vi "delay stage BBD301.vi"() -> ()   [LabVIEW 2024]
uses:
  C:/Users/QLM-CCD/Desktop/Pump probe/Kinesis/Thorlabs.MotionControl.Benchtop.BrushlessMotorCLI.dll
  Kinesis/Thorlabs.MotionControl.Benchtop.BrushlessMotorCLI.dll
  C:/Users/QLM-CCD/Desktop/Pump probe/Kinesis/Thorlabs.MotionControl.Controls.dll
  Kinesis/Thorlabs.MotionControl.Controls.dll
panel:
  in  "end poisition (mm)":dbl
  in  "stop":bool
  out "Position (micrometer)":i32
  in  "BenchtopBrushlessControl":refnum<k24>(container)
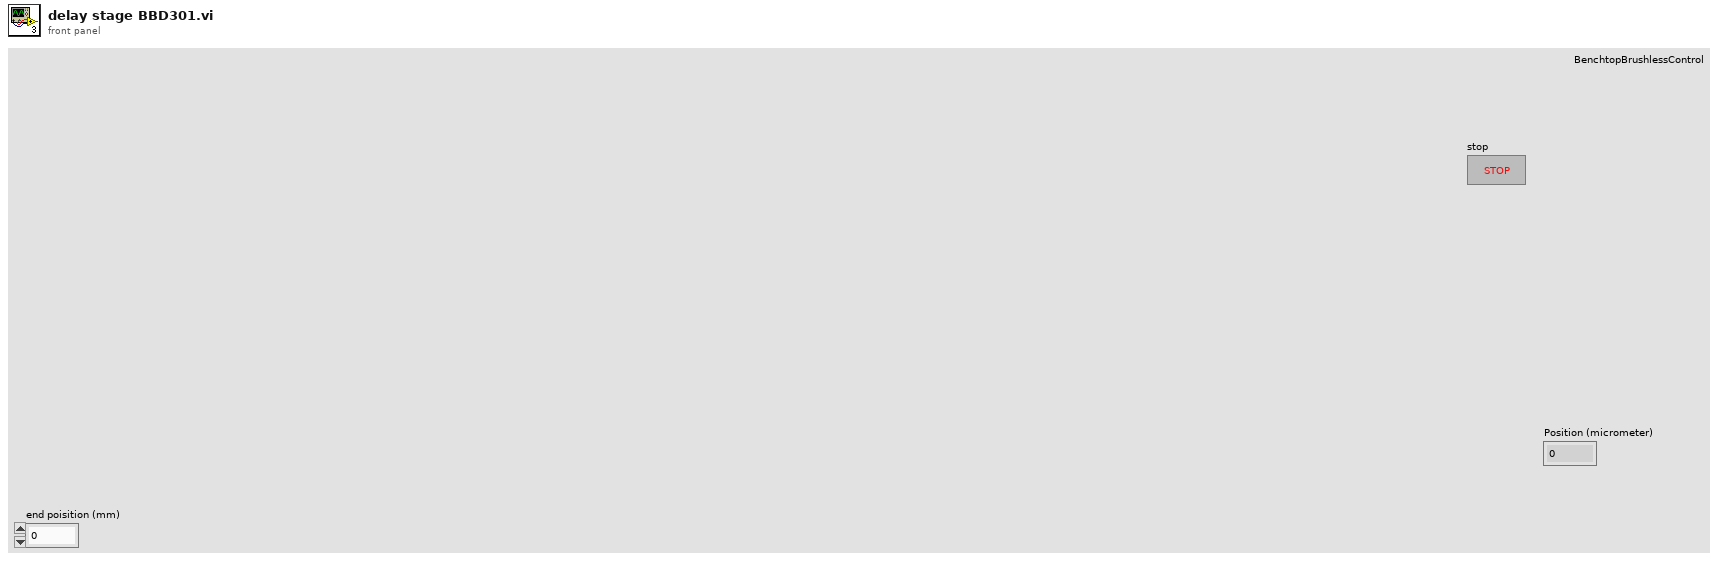
[diagram p1: front panel]
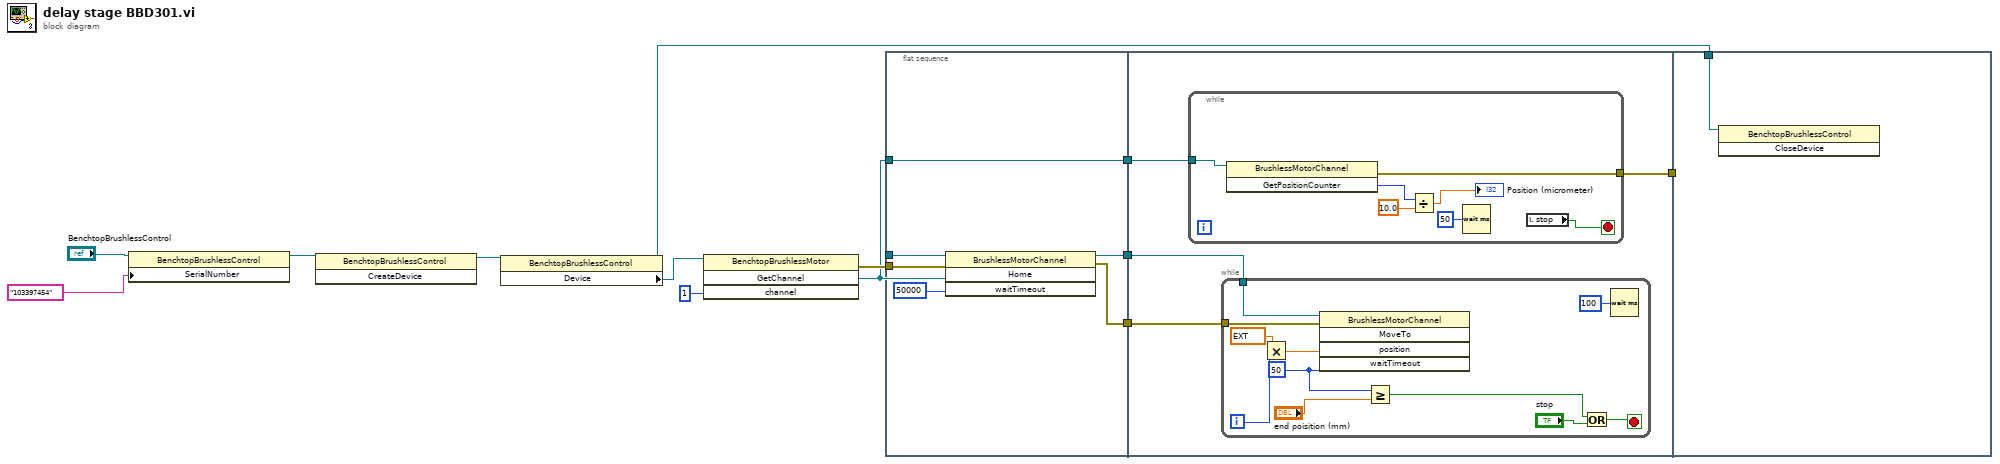
[diagram p0: block diagram]
diagram:
  n1 = property class="BenchtopBrushlessControl"(reference="BenchtopBrushlessControl", "SerialNumber"="103397454") -> (reference out=w9:refnum<k24>)  [unwired: 1 in, 1 out]
  n2 = invoke class="BenchtopBrushlessControl" method="CreateDevice"(reference=w9) -> (reference out=w5:refnum<k24>)  [unwired: 2 in, 2 out]
  n3 = property class="BenchtopBrushlessControl"(reference=w5) -> (reference out=w2:refnum<k24>, "Device"=w3:refnum<k24>)  [unwired: 1 in, 1 out]
  n4 = invoke class="BenchtopBrushlessMotor" method="GetChannel"(reference=w3, "channel"=i16 1) -> (error out=w6:errorcluster, "GetChannel"=w4:refnum<k24>)  [unwired: 2 in, 2 out]
  n5 = flat-sequence {
    tunnel: w4 -> [w19]
    tunnel: [w17] -> w13
    tunnel: w6 -> [w16]
    tunnel: [w15] -> w12
    tunnel: w4 -> [w14]
    tunnel: [w14] -> w11
    tunnel: w13 -> [w23]
    tunnel: w12 -> [w22]
    tunnel: w11 -> [w21]
    tunnel: [w20] -> w10
    tunnel: w10 -> [_]
    tunnel: w2 -> [w42]
    frame #0 {
      n6 = invoke class="BrushlessMotorChannel" method="Home"(reference=w19, error in=w16, "waitTimeout"=50000) -> (reference out=w17:refnum<k24>, error out=w15:errorcluster)  [unwired: 1 in, 2 out]
    }
    frame #1 {
      n7 = while {
        tunnel: w21 -> [w26]
        tunnel: [w24] -> w20
        stop <- w25 stop-if-true
        n8 = invoke class="BrushlessMotorChannel" method="GetPositionCounter"(reference=w26) -> (error out=w24:errorcluster, "GetPositionCounter"=w29:i32)  [unwired: 2 in, 1 out]
        n9 = Divide(x=w29, y=10.0) -> (x/y=→"Position (micrometer)":dbl)
        n10 = Wait (ms)(milliseconds to wait=u32 50) -> ()  [unwired: 1 out]
        n11 = local read "stop"() -> (w25:bool)
      }
      n12 = while {
        tunnel: w23 -> [w41]
        tunnel: w22 -> [w32]
        i -> [w38]
        stop <- w34 stop-if-true
        w35 = 50 ("waitTimeout")
        n13 = Multiply(x=ext 0.0001, y=w38) -> (x*y=w40:ext)
        n14 = invoke class="BrushlessMotorChannel" method="MoveTo"(reference=w41, error in=w32, "position"=w40, "waitTimeout"=w35) -> ()  [unwired: 1 in, 5 out]
        n15 = Greater Or Equal?(x=w35, y="end poisition (mm)") -> (x >= y?=w33:bool)
        n16 = Or(x=w33, y="stop") -> (x .or. y?=w34:bool)
        n17 = Wait (ms)(milliseconds to wait=u32 100) -> ()  [unwired: 1 out]
      }
    }
    frame #2 {
      n18 = invoke class="BenchtopBrushlessControl" method="CloseDevice"(reference=w42) -> ()  [unwired: 2 in, 3 out]
    }
  }
